vi "曲线去两端.vi"(11 "曲线In":cluster{"X":dbl[], "Y":dbl[]}[](array[cluster])) -> (2 "启动曲线":cluster{"X":dbl[], "Y":dbl[]}[](array[cluster]), 3 "曲线Out":cluster{"X":dbl[], "Y":dbl[]}[](array[cluster]))   [LabVIEW 2020]
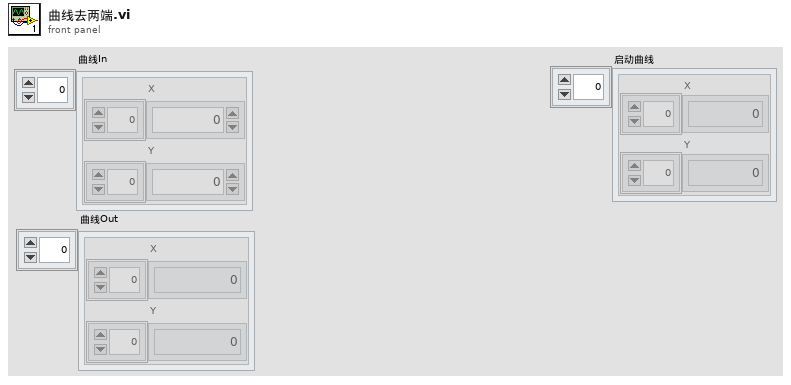
[diagram p1: front panel]
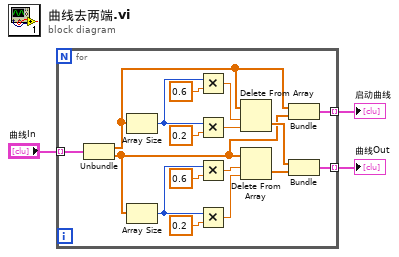
[diagram p0: block diagram]
diagram:
  n1 = for {
    tunnel: "曲线In" -> [w17] mode=indexing
    tunnel: [w11] -> w2 mode=indexing
    tunnel: [w8] -> w1 mode=indexing
    n2 = Unbundle(w17) -> ("X"=w5:dbl[], "Y"=w4:dbl[])
    n3 = Array Size(array=w5) -> (size(s)=w19:i32)
    n4 = Array Size(array=w4) -> (size(s)=w15:i32)
    n5 = Multiply(x=w19, y=0.6) -> (x*y=w10:dbl)
    n6 = Multiply(x=w19, y=0.2) -> (x*y=w9:dbl)
    n7 = Multiply(x=w15, y=0.6) -> (x*y=w6:dbl)
    n8 = Multiply(x=w15, y=0.2) -> (x*y=w7:dbl)
    n9 = Delete From Array ("删除数组元素")(array=w5, length=w10, index=w9) -> (deleted portion=w13:dbl[])  [unwired: 1 out]
    n10 = Delete From Array(array=w4, length=w6, index=w7) -> (deleted portion=w12:dbl[])  [unwired: 1 out]
    n11 = Bundle("X"=w5, "Y"=w4) -> (w8:cluster{"X":dbl[], "Y":dbl[]})  [unwired: 1 in]
    n12 = Bundle("X"=w13, "Y"=w12) -> (w11:cluster{"X":dbl[], "Y":dbl[]})  [unwired: 1 in]
  }
  "曲线Out" <- w2
  "启动曲线" <- w1
